vi "Save.vi"(8 "error in (no error)":errorcluster, 11 "PackageAbstract in":refnum<class "PackageAbstract.lvclass">) -> (0 "error out":errorcluster, 3 "PackageAbstract out":refnum<class "PackageAbstract.lvclass">)   [LabVIEW 2020, in "GPack.lvlib" / "PackageAbstract.lvclass"]
uses:
  PackageAbstract.lvclass
  GPack File/GPack File.lvclass
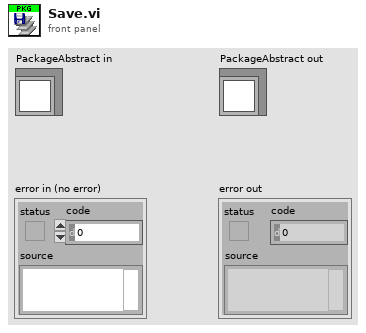
[diagram p1: front panel]
types:
  T1 = typedef "GPack.lvlib/Package Info.ctl" = cluster{"Name":string, "Type":string, "Host":string, "Path":string, "Branch":string, "Version":string}
  T2 = typedef "GPack.lvlib/Dependency.ctl" = cluster{"Info":T1, "Path":path}
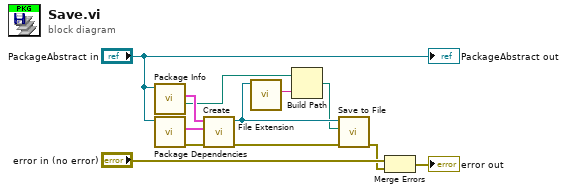
[diagram p0: block diagram]
diagram:
  n1 = call-dynamic "Package Info.vi"("Package in"="PackageAbstract in") -> ("Folder"=w6:path, "Package Info"=w9:T1)  [unwired: 8 in, 1 out]
  n2 = call-dynamic "Package Dependencies.vi"("PackageAbstract in"="PackageAbstract in") -> ("error out"=w11:errorcluster, "Dependencies"=w10:T2[])  [unwired: 9 in]
  n3 = call "Create.vi"("error in (no error)"=w11, "Dependencies"=w10, "Package Info"=w9) -> ("error out"=w5:errorcluster, "GPack File out"=w4:refnum<class "GPack File.lvclass">)  [unwired: 7 in]
  n4 = call-dynamic "File Extension.vi"("GPack File in"=w4) -> ("File Extension"=w7:string)  [unwired: 9 in, 1 out]
  n5 = Build Path(base path=w6, name or relative path=w7) -> (appended path=w3:path)
  n6 = call-dynamic "Save to File.vi"("error in (no error)"=w5, "Path"=w3, "GPack File in"=w4) -> ("error out"=w1:errorcluster)  [unwired: 7 in, 1 out]
  n7 = Merge Errors("error in (no error)", w1) -> (→"error out":errorcluster)
  "PackageAbstract out" <- "PackageAbstract in"
